vi "VescSetRpm.vi"(11 "RPM":u16) -> ()   [LabVIEW 2019]
uses:
  <vilib>/myRIO/Instrument Drivers/Onboard IO/UART/typedef/VISA Configuration.ctl
  <vilib>/Instr/_visa.llb/VISA Configure Serial Port (Instr).vi
  <vilib>/myRIO/Express VI/Onboard IO/UART/UART Express VI.xnode
  <vilib>/myRIO/Instrument Drivers/Onboard IO/UART/UART.lvlib
  usr/local/lib/libvescEncoder.so
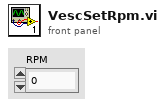
[diagram p1: front panel]
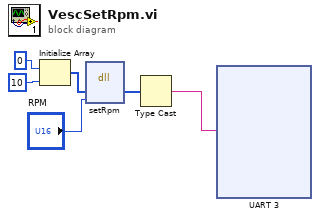
[diagram p0: block diagram]
diagram:
  n1 = Initialize Array(0, 10) -> (w3:i32[])
  n2 = dll-call lib="usr/local/lib/libvescEncoder.so" fn="setRpm"("array"=w3, "rpm"="RPM") -> ("array"=w2:u8[])  [unwired: 5 in, 2 out]
  n3 = Type Cast(x=w2) -> (*(type *) &x=w6:string)  [unwired: 1 in]
  n4 = xnode "UART 3"("Characters to Write"=w6) -> ()  [unwired: 1 in, 2 out]
